vi "exercise7.vi"() -> ()   [LabVIEW 2020]
uses:
  rappg_lab3/Control 1.ctl
  <vilib>/measure/mascope.llb/Amplitude and Levels 1 chan.vi
  <vilib>/Analysis/NI_AALBase.lvlib
  <vilib>/measure/NI_MAPro.lvlib
panel:
  out "high state level":dbl format="%.2g"
  out "amplitude measurement":dbl format="%.2p"
  in  "state settings":T1={"method"=enum."auto select", "histogram size"=256, "histogram method"=enum."mode", "reserved"=1.0} {"reserved" format="%0.2f"}
  in  "amplitude":dbl=1.0 format="%0.2f"
  in  "stop":bool
  in  "Analyze Data":bool
  in  "Acquire Data":bool
  out "Waveform Graph":dbl[](graph)
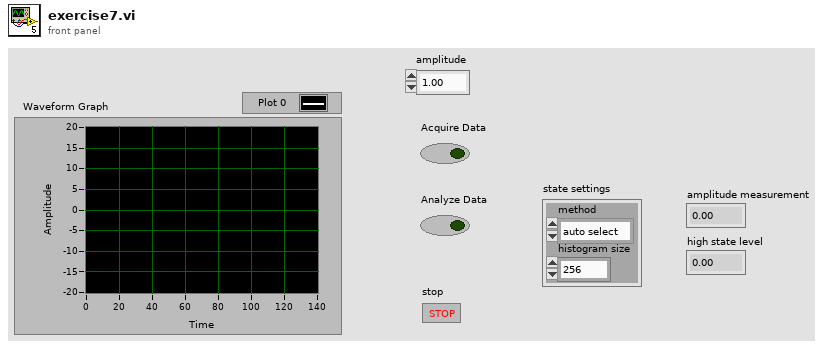
[diagram p1: front panel]
types:
  T1 = cluster{"method":enum32{"histogram", "peak", "auto select"}, "histogram size":i32, "histogram method":enum16{"mode"}, "reserved":dbl}
  T2 = typedef "Control 1.ctl" = enum16{"Initialize", "Stop", "Check for UI Events", "Acquire Data", "Analyze Data"}
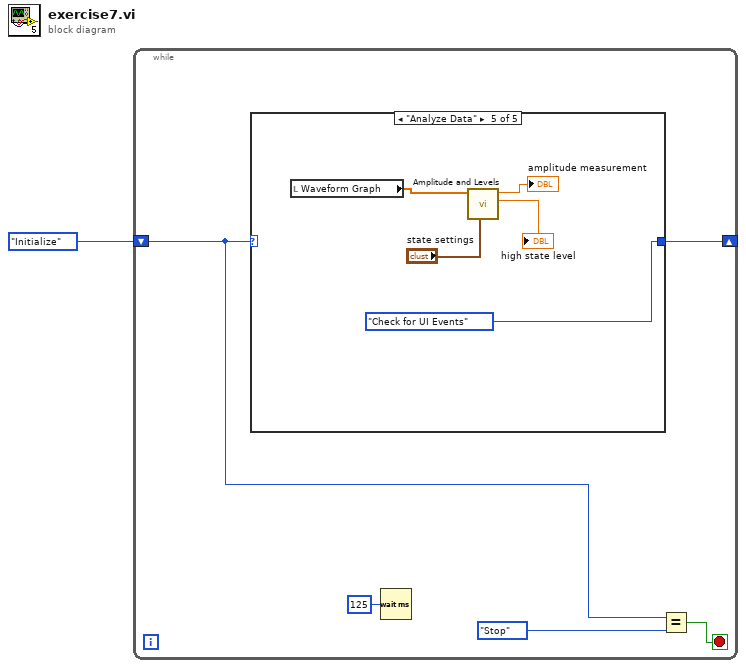
[diagram p0: block diagram]
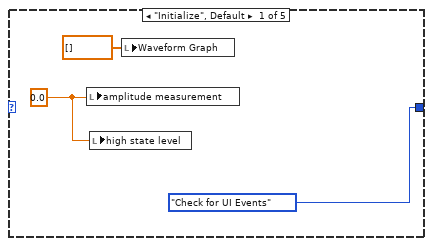
[diagram p2: hidden frame]
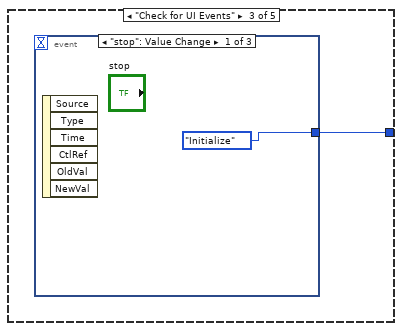
[diagram p4: hidden frame]
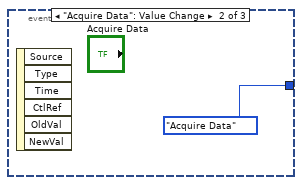
[diagram p5: hidden frame]
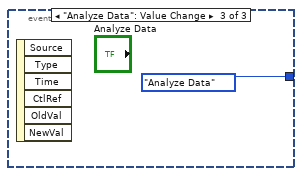
[diagram p6: hidden frame]
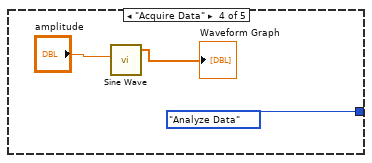
[diagram p7: hidden frame]
diagram:
  n1 = while {
    shift-right: [w5] -> _
    shift-left: Control_1."Initialize" -> [w4]
    stop <- w6 stop-if-true
    n2 = case shown="\"Analyze Data\"" w4 {
      tunnel: [Control_1."Check for UI Events" _ w10 Control_1."Analyze Data" Control_1."Check for UI Events"] -> w5
      frame "Initialize", Default {
        w8 = 0.0 ("amplitude measurement")
        n3 = local write "amplitude measurement"(w8) -> ()
        n4 = local write "high state level"(w8) -> ()
        n5 = local write "Waveform Graph"(dbl[] [] ("Waveform Graph")) -> ()
      }
      frame "Stop" {
      }
      frame "Check for UI Events" {
        n6 = event shown="[0] \"stop\": Value Change" {
          selector: _ -> [_ _ _]
          dyn-events: _ -> [_ _ _]
          timeout: _ -> [_ _ _]
          tunnel: [Control_1."Initialize" Control_1."Acquire Data" Control_1."Analyze Data"] -> w10
          event "stop": Value Change {
            n7 = event-data() -> ()  [unwired: 1 in, 6 out]
          }
          event "Acquire Data": Value Change {
            n8 = event-data() -> ()  [unwired: 1 in, 6 out]
          }
          event "Analyze Data": Value Change {
            n9 = event-data() -> ()  [unwired: 1 in, 6 out]
          }
        }
      }
      frame "Acquire Data" {
        n10 = call <vilib>:"Sine Wave.vi"("amplitude"="amplitude") -> ("sine wave"=→"Waveform Graph":dbl[])  [unwired: 4 in, 2 out]
      }
      frame "Analyze Data" {
        n11 = local read "Waveform Graph"() -> (w21:dbl[])
        n12 = call-poly <vilib>:"Amplitude and Levels.vi"("state settings"="state settings", "signal in"=w21) -> ("high state level"=→"high state level":dbl, "amplitude"=→"amplitude measurement":dbl)  [unwired: 6 in, 2 out]
      }
    }
    n13 = Wait (ms)(milliseconds to wait=u32 125) -> ()  [unwired: 1 out]
    n14 = Equal?(x=w4, y=Control_1."Stop") -> (x = y?=w6:bool)
  }
